vi "SimulatedPeak.vi"(0 "Time Length":dbl=20.0, 1 "Sampling Interval":dbl=0.005, 2 "offset":dbl=1.0, 3 "Width":dbl=1.0, 4 "Center":dbl=10.0, 5 "Noise Level":dbl=0.02, 8 "Amplitude":dbl=4.0) -> (7 "Simulated Peak":waveform(dbl))   [LabVIEW 2020]
doc: "This VI can be used to simulate Gaussian peak."
uses:
  <vilib>/Analysis/NI_AALBase.lvlib
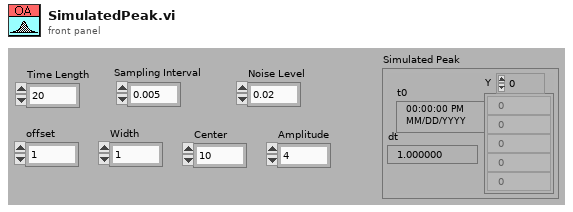
[diagram p1: front panel]
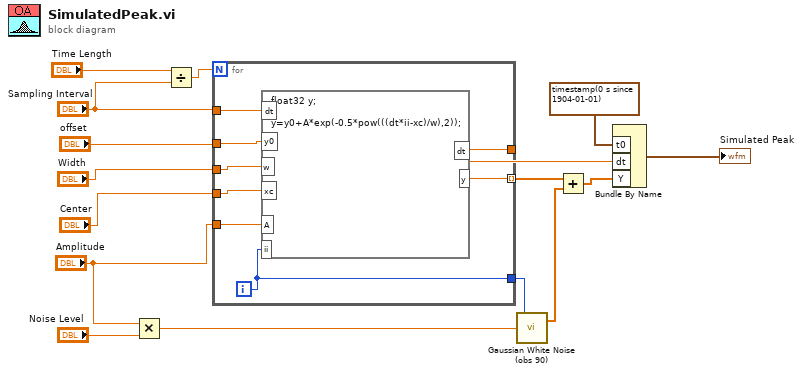
[diagram p0: block diagram]
diagram:
  n1 = Multiply(x="Amplitude", y="Noise Level") -> (x*y=w16:dbl)
  n2 = Divide(x="Time Length", y="Sampling Interval") -> (x/y=w4:dbl)
  n3 = for {
    N: w4 -> [_]
    tunnel: [w24] -> w11 mode=indexing
    tunnel: [w23] -> w2
    tunnel: "Amplitude" -> [w22]
    tunnel: "Width" -> [w21]
    tunnel: "Center" -> [w20]
    tunnel: "Sampling Interval" -> [w19]
    tunnel: "offset" -> [w18]
    tunnel: [w17] -> w9
    i -> [w17]
    n4 = formula code="float32 y; \n\ny=y0+A*exp(-0.5*pow(((dt*ii-xc)/w),2));"("xc"=w20, "A"=w22, "w"=w21, "ii"=w17, "dt"=w19, "y0"=w18) -> ("y"=w24:sgl, "dt"=w23:dbl)
  }
  n5 = call <vilib>:"Gaussian White Noise (obs 90).vi"("standard deviation"=w16, "samples"=w9) -> ("Gaussian noise pattern"=w10:dbl[])  [unwired: 1 in, 1 out]
  n6 = Add(x=w11, y=w10) -> (x+y=w12:dbl[])
  n7 = Bundle By Name("t0"=timestamp(0 s since 1904-01-01), "dt"=w2, "Y"=w12) -> (→"Simulated Peak":waveform(dbl))  [unwired: 1 in]
